vi "AO.vi"(8 "error in":errorcluster, 10 "AO Array":waveform(dbl)[](array[waveform]), 11 "AO Task":refnum<k21>[](array[refnum])) -> (0 "error out":errorcluster)   [LabVIEW 2016, in "LockinDAQ.lvclass"]
uses:
  LockinDAQ.lvclass
  <vilib>/DAQmx/write.llb/DAQmx Write (Analog 1D Wfm NChan NSamp).vi
  <vilib>/DAQmx/miscellaneous.llb/DAQmx Fill In Error Info.vi
panel:
  out "number of samples written per channel 4":u32
  out "number of samples written per channel 3":u32
  out "number of samples written per channel 2":u32
  out "number of samples written per channel 1":u32
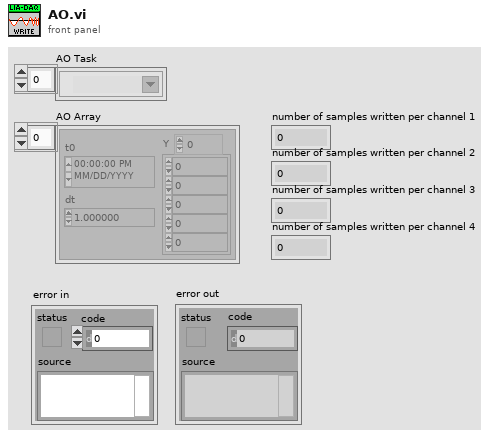
[diagram p1: front panel]
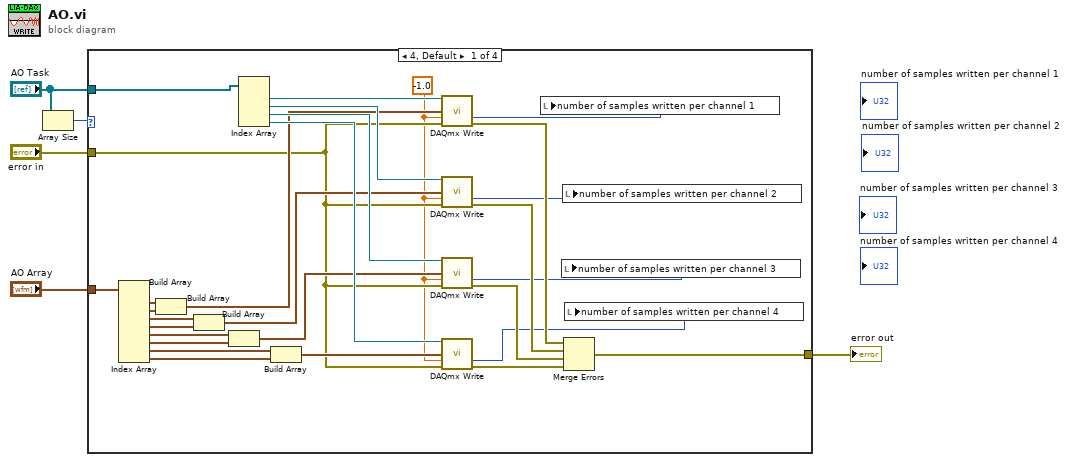
[diagram p0: block diagram]
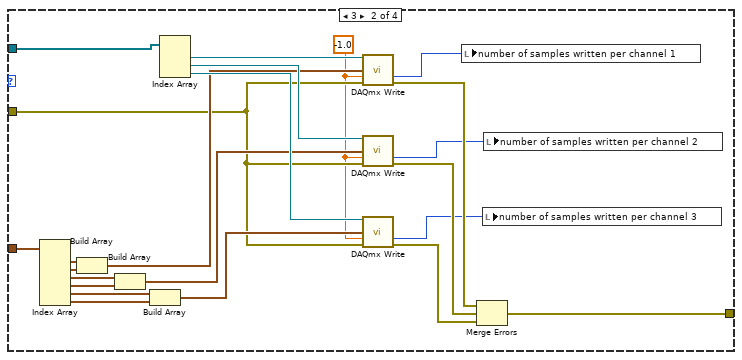
[diagram p2: hidden frame]
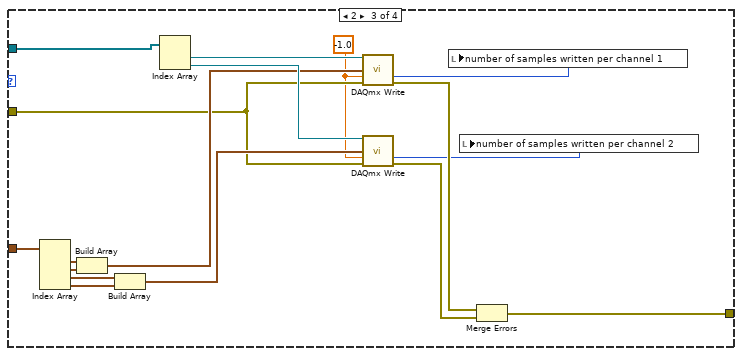
[diagram p3: hidden frame]
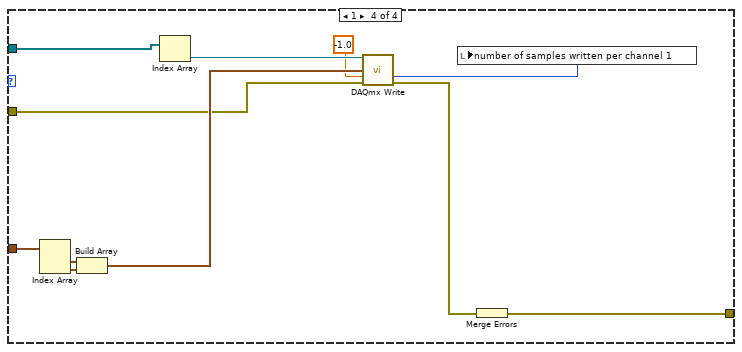
[diagram p4: hidden frame]
diagram:
  n1 = Array Size(array="AO Task") -> (size(s)=w1:i32)
  n2 = case shown="4, Default" w1 {
    tunnel: "AO Array" -> [w33 w57 w74 w85]
    tunnel: "AO Task" -> [w32 w56 w73 w84]
    tunnel: "error in" -> [w16 w43 w64 w79]
    tunnel: [w11 w39 w62 w77] -> w3
    frame 4, Default {
      w10 = -1.0 ("timeout")
      n3 = Index Array(array=w33) -> (element #1=w27:waveform(dbl), element #2=w26:waveform(dbl), element #3=w25:waveform(dbl), element #4=w24:waveform(dbl), element #5=w23:waveform(dbl), element #6=w22:waveform(dbl), element #7=w21:waveform(dbl), element #8=w20:waveform(dbl))  [unwired: 8 in]
      n4 = Build Array(w27, w26) -> (w19:waveform(dbl)[])
      n5 = Build Array(w25, w24) -> (w18:waveform(dbl)[])
      n6 = Build Array(w23, w22) -> (w17:waveform(dbl)[])
      n7 = Index Array(array=w32) -> (element #1=w31:refnum<k21>, element #2=w30:refnum<k21>, element #3=w29:refnum<k21>, element #4=w28:refnum<k21>)  [unwired: 4 in]
      n8 = Build Array(w21, w20) -> (w34:waveform(dbl)[])
      n9 = call-poly <vilib>:"DAQmx Write.vi"("task/channels in"=w31, "data"=w19, "timeout"=w10, "error in"=w16) -> ("number of samples written per channel"=w6:u32, "error out"=w12:errorcluster)  [unwired: 9 in, 1 out]
      n10 = call-poly <vilib>:"DAQmx Write.vi"("task/channels in"=w30, "data"=w18, "timeout"=w10, "error in"=w16) -> ("number of samples written per channel"=w7:u32, "error out"=w15:errorcluster)  [unwired: 9 in, 1 out]
      n11 = call-poly <vilib>:"DAQmx Write.vi"("task/channels in"=w29, "data"=w17, "timeout"=w10, "error in"=w16) -> ("number of samples written per channel"=w8:u32, "error out"=w14:errorcluster)  [unwired: 9 in, 1 out]
      n12 = call-poly <vilib>:"DAQmx Write.vi"("task/channels in"=w28, "data"=w34, "timeout"=w10, "error in"=w16) -> ("number of samples written per channel"=w9:u32, "error out"=w13:errorcluster)  [unwired: 9 in, 1 out]
      n13 = local write "number of samples written per channel 1"(w6) -> ()
      n14 = local write "number of samples written per channel 3"(w8) -> ()
      n15 = local write "number of samples written per channel 2"(w7) -> ()
      n16 = Merge Errors(w12, w15, w14, w13) -> (w11:errorcluster)
      n17 = local write "number of samples written per channel 4"(w9) -> ()
    }
    frame 3 {
      w38 = -1.0 ("timeout")
      n18 = Index Array(array=w57) -> (element #1=w52:waveform(dbl), element #2=w51:waveform(dbl), element #3=w50:waveform(dbl), element #4=w49:waveform(dbl), element #5=w48:waveform(dbl), element #6=w47:waveform(dbl))  [unwired: 6 in]
      n19 = Build Array(w52, w51) -> (w46:waveform(dbl)[])
      n20 = Build Array(w50, w49) -> (w45:waveform(dbl)[])
      n21 = Build Array(w48, w47) -> (w44:waveform(dbl)[])
      n22 = Index Array(array=w56) -> (element #1=w55:refnum<k21>, element #2=w54:refnum<k21>, element #3=w53:refnum<k21>)  [unwired: 3 in]
      n23 = call-poly <vilib>:"DAQmx Write.vi"("task/channels in"=w55, "data"=w46, "timeout"=w38, "error in"=w43) -> ("number of samples written per channel"=w37:u32, "error out"=w40:errorcluster)  [unwired: 9 in, 1 out]
      n24 = call-poly <vilib>:"DAQmx Write.vi"("task/channels in"=w54, "data"=w45, "timeout"=w38, "error in"=w43) -> ("number of samples written per channel"=w36:u32, "error out"=w42:errorcluster)  [unwired: 9 in, 1 out]
      n25 = call-poly <vilib>:"DAQmx Write.vi"("task/channels in"=w53, "data"=w44, "timeout"=w38, "error in"=w43) -> ("number of samples written per channel"=w35:u32, "error out"=w41:errorcluster)  [unwired: 9 in, 1 out]
      n26 = local write "number of samples written per channel 1"(w37) -> ()
      n27 = Merge Errors(w40, w42, w41) -> (w39:errorcluster)
      n28 = local write "number of samples written per channel 3"(w35) -> ()
      n29 = local write "number of samples written per channel 2"(w36) -> ()
    }
    frame 2 {
      w61 = -1.0 ("timeout")
      n30 = Index Array(array=w74) -> (element #1=w70:waveform(dbl), element #2=w69:waveform(dbl), element #3=w68:waveform(dbl), element #4=w67:waveform(dbl))  [unwired: 4 in]
      n31 = Build Array(w70, w69) -> (w66:waveform(dbl)[])
      n32 = Build Array(w68, w67) -> (w65:waveform(dbl)[])
      n33 = Index Array(array=w73) -> (element #1=w72:refnum<k21>, element #2=w71:refnum<k21>)  [unwired: 2 in]
      n34 = call-poly <vilib>:"DAQmx Write.vi"("task/channels in"=w72, "data"=w66, "timeout"=w61, "error in"=w64) -> ("number of samples written per channel"=w58:u32, "error out"=w63:errorcluster)  [unwired: 9 in, 1 out]
      n35 = call-poly <vilib>:"DAQmx Write.vi"("task/channels in"=w71, "data"=w65, "timeout"=w61, "error in"=w64) -> ("number of samples written per channel"=w59:u32, "error out"=w60:errorcluster)  [unwired: 9 in, 1 out]
      n36 = local write "number of samples written per channel 1"(w58) -> ()
      n37 = local write "number of samples written per channel 2"(w59) -> ()
      n38 = Merge Errors(w63, w60) -> (w62:errorcluster)
    }
    frame 1 {
      n39 = Index Array(array=w85) -> (element #1=w82:waveform(dbl), element #2=w81:waveform(dbl))  [unwired: 2 in]
      n40 = Build Array(w82, w81) -> (w80:waveform(dbl)[])
      n41 = Index Array(array=w84) -> (element=w83:refnum<k21>)  [unwired: 1 in]
      n42 = call-poly <vilib>:"DAQmx Write.vi"("task/channels in"=w83, "data"=w80, "timeout"=-1.0, "error in"=w79) -> ("number of samples written per channel"=w75:u32, "error out"=w78:errorcluster)  [unwired: 9 in, 1 out]
      n43 = local write "number of samples written per channel 1"(w75) -> ()
      n44 = Merge Errors(w78) -> (w77:errorcluster)
    }
  }
  "error out" <- w3
